vi "NotchCoeffMultiChanQTemplate.vi"(0 "notch frequency":dbl=2.0 format="%#_6p", 5 "Q factor":dbl=20.0 format="%#_6p", 9 "sample rate":dbl=50000.0 format="%#_6p", 11 "error in (no error)":errorcluster, 12 "channel index":u16) -> (4 "configuration":T1, 15 "error out":errorcluster)   [LabVIEW 2017, in "NI_FpgaMspHost.lvlib"]
doc: "This VI designs a Butterworth filter, then quantizes and formats the coefficients into 32-bit integers for use by the Butterworth Filter VI on the FPGA.\n\nThe user is responsible for ensuring that the configuration is valid. The following restrictions apply:\nCutoff frequency must meet Nyquist criterion.\nMultichannel filters are restricted to 2nd order.\nFilter order and type cannot be changed at run-time."
uses:
  <vilib>/rvi/Analysis/host/Public/NI_FpgaMspHost.lvlib
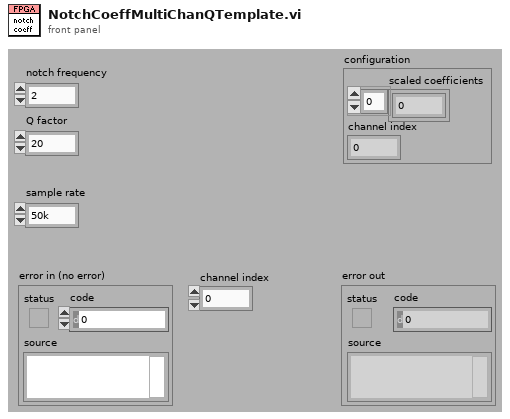
[diagram p1: front panel]
types:
  T1 = cluster{"scaled coefficients":i32[], "channel index":u16}
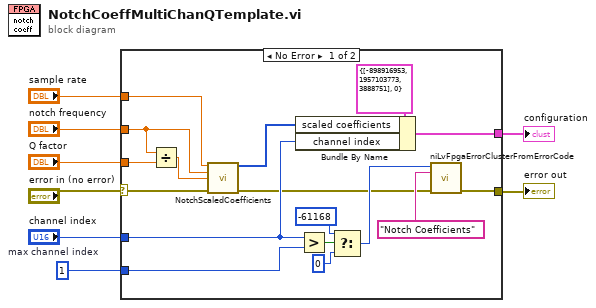
[diagram p0: block diagram]
diagram:
  w3 = u16 1  # max channel index
  n1 = case shown="No Error" "error in (no error)" {
    selector: "error in (no error)" -> [w13 w26]
    tunnel: "sample rate" -> [w25 _]
    tunnel: [w22 _] -> w7
    tunnel: "notch frequency" -> [w21 _]
    tunnel: "Q factor" -> [w20 _]
    tunnel: "channel index" -> [w15 _]
    tunnel: w3 -> [w14 _]
    tunnel: [w9 w26] -> w2
    frame No Error {
      n2 = Divide(x=w21, y=w20) -> (x/y=w19:dbl)
      n3 = call <vilib>:"NotchScaledCoefficients.vi"("sample rate (S/s)"=w25, "notch frequency (Hz)"=w21, "notch width (Hz)"=w19, "error in (no error)"=w13) -> ("scaled coefficients"=w23:i32[], "error out"=w10:errorcluster)  [unwired: 2 in, 8 out]
      n4 = Bundle By Name(cluster=T1 {"scaled coefficients"=[-898916953, 1957103773, 3888751], "channel index"=0} ("scaled coefficients"), "scaled coefficients"=w23, "channel index"=w15) -> (w22:T1)
      n5 = Greater?(x=w15, y=w14) -> (0:w18:bool)
      n6 = Select(t=-61168, s=w18, f=0 ("Error Code")) -> (s? t:f=w11:i32)
      n7 = call <vilib>:"niLvFpgaErrorClusterFromErrorCode.vi"("error code"=w11, "function name"="Notch Coefficients" ("subVI name"), "error in"=w10) -> ("error out"=w9:errorcluster)  [unwired: 4 in, 8 out]
    }
    frame Error {
    }
  }
  "error out" <- w2
  "configuration" <- w7
